vi "Logging.vi"(8 "error in (no error)":errorcluster, 11 "Node Ptr":T2 format="%.0x") -> (0 "error out":errorcluster)   [LabVIEW 2020, in "Ballard MIL-STD-1553 System Explorer.lvlib" / "Implementation.lvlib"]
uses:
  Implementation.lvlib
  <vilib>/NI VeriStand/Custom Device API/Custom Device Item Ref.ctl
  Shared/Data Word Format.ctl
  <vilib>/NI VeriStand/Custom Device API/Custom Device API.lvlib
  Scripting/Ballard MIL-STD-1553 Scripting.lvlib
panel:
  in  "Data Word Format":T1
  in  "Timestamp Filename":bool
  in  "File Name":string
  out "Example Log File Path":string
  in  "Enable Logging":bool
  in  "Log Directory":string
  in  "SHDocVw.IWebBrowser":refnum<k7>(container)
  in  "General Header":cluster{"Section Name":string}={"Section Name"="Ballard MIL-STD-1553 - Logging"}
  in  "Description":string
  out "Name":string
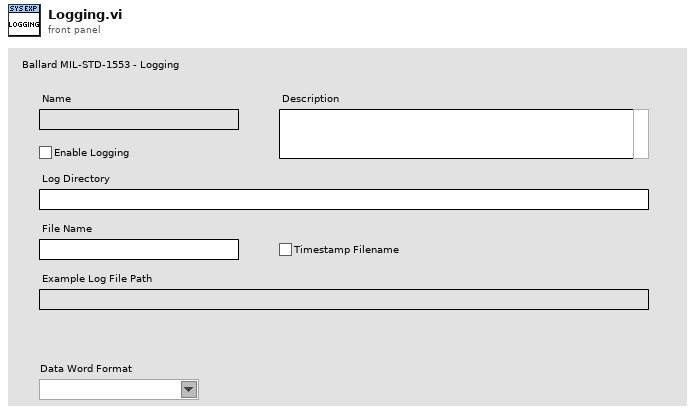
[diagram p1: front panel]
types:
  T1 = typedef "Data Word Format.ctl" = string
  T2 = typedef "Custom Device API.lvlib/Custom Device Item Ref.ctl" = u64
  T3 = typedef "Custom Device API.lvlib/Custom Device Item Info.ctl" = cluster{"Name":string, "Is Channel":bool, "GUID":string, "Is Waveform":bool}
  T4 = typedef "Custom Device API.lvlib/Custom Device Commands.ctl" = enum16{"Default", "Item renamed", "Shutdown", "Dynamic button pressed"}
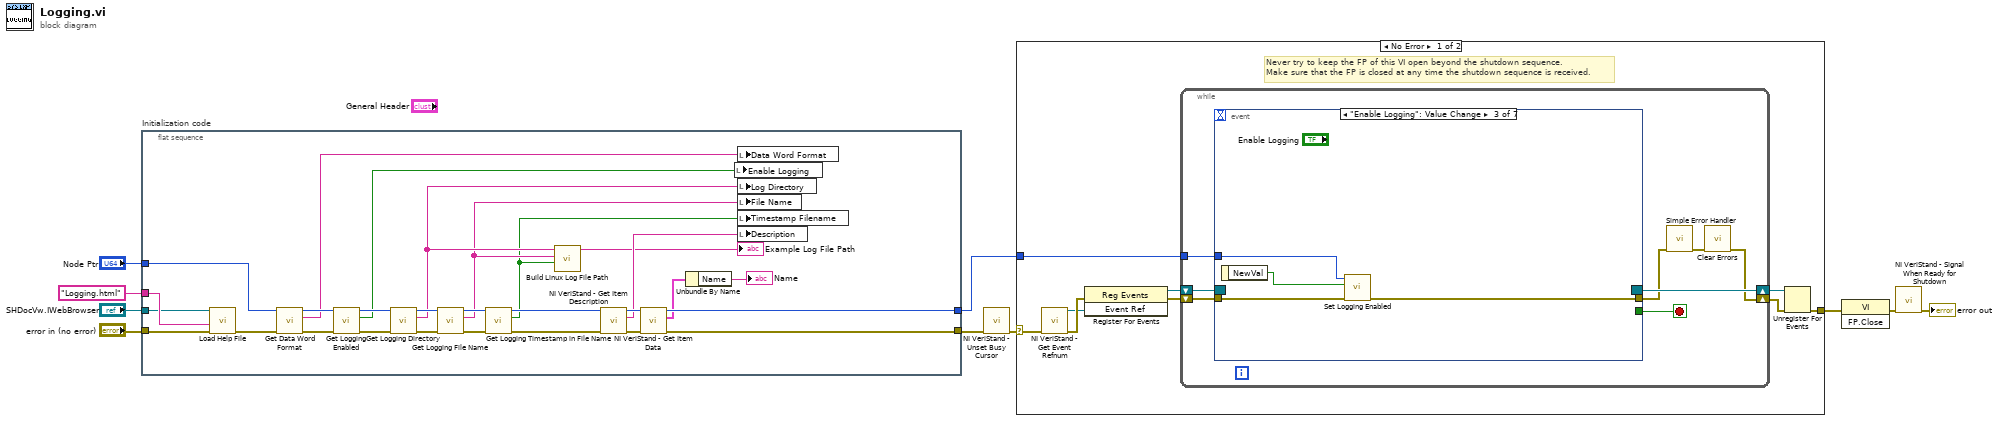
[diagram p0: block diagram]
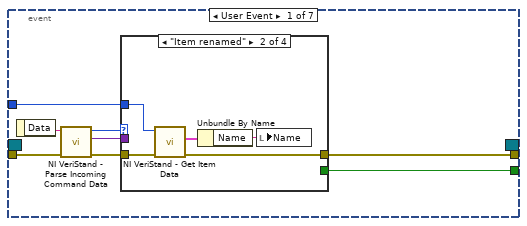
[diagram p2: hidden frame]
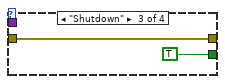
[diagram p4: hidden frame]
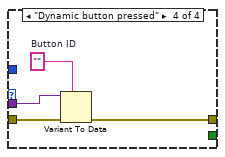
[diagram p5: hidden frame]
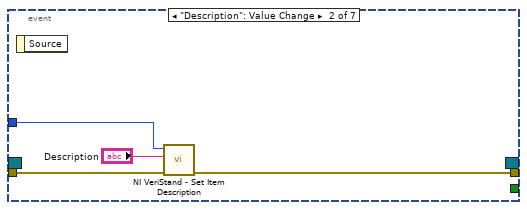
[diagram p6: hidden frame]
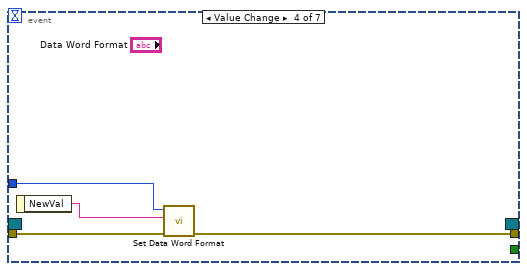
[diagram p7: hidden frame]
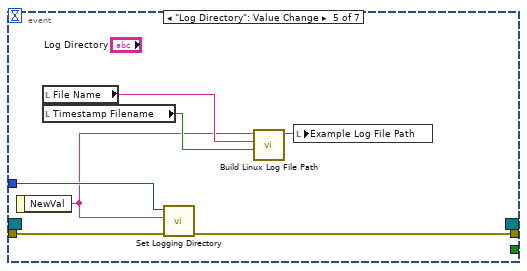
[diagram p8: hidden frame]
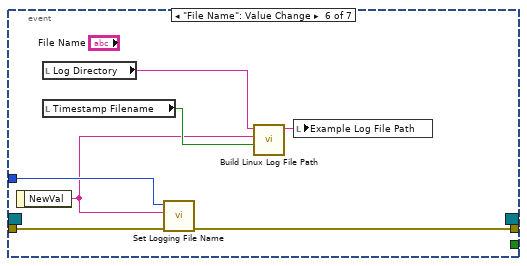
[diagram p9: hidden frame]
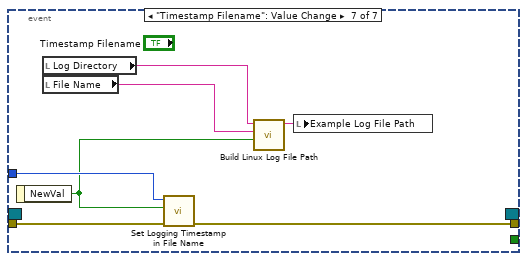
[diagram p10: hidden frame]
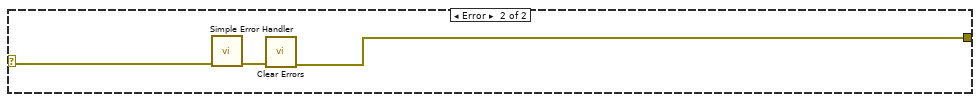
[diagram p11: hidden frame]
diagram:
  n1 = flat-sequence "Initialization code" {
    tunnel: "error in (no error)" -> [w32]
    tunnel: "Node Ptr" -> [w23]
    tunnel: [w34] -> w6
    tunnel: [w38] -> w3
    tunnel: "SHDocVw.IWebBrowser" -> [w30]
    tunnel: "Logging.html" ("CD_CHM_Section") -> [w31]
    frame #0 {
      n2 = call "Load Help File.vi"("error in (no error)"=w32, "HTML File to Load"=w31, "Browser"=w30) -> ("error out"=w28:errorcluster)  [unwired: 8 in]
      n3 = call "Get Data Word Format.vi"("error in"=w28, "logging in"=w23) -> ("error out"=w24:errorcluster, "data word format"=w21:T1, "logging out"=w22:T2)  [unwired: 7 in]
      n4 = call "Get Logging Enabled.vi"("error in"=w24, "logging in"=w22) -> ("error out"=w27:errorcluster, "logging enabled"=w25:bool, "logging out"=w26:T2)  [unwired: 7 in]
      n5 = call "Get Logging Directory.vi"("error in"=w27, "logging in"=w26) -> ("error out"=w19:errorcluster, "directory"=w13:string, "logging out"=w20:T2)  [unwired: 7 in]
      n6 = call "Get Logging File Name.vi"("error in"=w19, "logging in"=w20) -> ("error out"=w18:errorcluster, "file name"=w12:string, "logging out"=w17:T2)  [unwired: 7 in]
      n7 = call "Get Logging Timestamp in File Name.vi"("error in"=w18, "logging in"=w17) -> ("error out"=w16:errorcluster, "timestamp in file name"=w11:bool, "logging out"=w15:T2)  [unwired: 7 in]
      n8 = call "Build Linux Log File Path.vi"("Timestamp"=w11, "Name"=w12, "Log File Directory"=w13) -> ("Log File Path"=→"Example Log File Path":string)  [unwired: 7 in, 1 out]
      n9 = call <vilib>:"NI VeriStand - Get Item Description.vi"("error in (no error)"=w16, "Item Ref in"=w15) -> ("error out"=w36:errorcluster, "Description"=w33:string, "Item Ref out"=w37:T2)  [unwired: 7 out]
      n10 = call <vilib>:"NI VeriStand - Get Item Data.vi"("error in (no error)"=w36, "Item Ref in"=w37) -> ("error out"=w34:errorcluster, "Item Info"=w35:T3, "Item Ref out"=w38:T2)  [unwired: 7 out]
      n11 = Unbundle By Name(w35) -> ("Name"=→"Name":string)
      n12 = local write "Enable Logging"(w25) -> ()
      n13 = local write "Data Word Format"(w21) -> ()
      n14 = local write "Log Directory"(w13) -> ()
      n15 = local write "File Name"(w12) -> ()
      n16 = local write "Timestamp Filename"(w11) -> ()
      n17 = local write "Description"(w33) -> ()
    }
  }
  n18 = call <vilib>:"NI VeriStand - Unset Busy Cursor.vi"("error in (no error)"=w6) -> ("error out"=w5:errorcluster)  [unwired: 10 out]
  n19 = case shown="No Error" w5 {
    selector: w5 -> [w39 w111]
    tunnel: [w44 w109] -> w10
    tunnel: w3 -> [w40 _]
    frame No Error {
      # "Never try to keep the FP of this VI open beyond the shutdown sequence.\nMake sure that the FP is closed at any time the shutdown sequence is received."
      n20 = call <vilib>:"NI VeriStand - Get Event Refnum.vi"("error in (no error)"=w39) -> ("error out"=w47:errorcluster, "Event Ref"=w43:refnum<user-event>)  [unwired: 9 out]
      n21 = register-events(error in=w47, w43) -> (reference out=w41:refnum<event-registration>, error out=w42:errorcluster)  [unwired: 1 in]
      n22 = while {
        tunnel: w40 -> [w51]
        shift-right: [w48] -> w45
        shift-left: w42 -> [w54]
        shift-right: [w55] -> w46
        shift-left: w41 -> [w53]
        stop <- w52 stop-if-true
        n23 = event shown="[2] \"Enable Logging\": Value Change" {
          selector: w53 -> [_ _ _ _ _ _ _]
          dyn-events: [_ _ _ _ _ _ _] -> w55
          timeout: _ -> [_ _ _ _ _ _ _]
          tunnel: w54 -> [w63 w78 w83 w86 w94 w101 w108]
          tunnel: [w59 _ _ _ _ _ _] -> w52
          tunnel: [w58 w77 w82 w87 w92 w100 w107] -> w50
          tunnel: w51 -> [w57 w79 w81 w85 w93 w99 w106]
          event User Event {
            n24 = event-data() -> ("Data"=w62:string)  [unwired: 1 out]
            n25 = call <vilib>:"NI VeriStand - Parse Incoming Command Data.vi"("error in (no error)"=w63, "Incoming data"=w62) -> ("error out"=w61:errorcluster, "Outgoing data"=w56:variant, "Action"=w60:T4)  [unwired: 7 out]
            n26 = case shown="\"Item renamed\"" w60 {
              tunnel: w61 -> [w64 w69 w70 w75]
              tunnel: [_ _ TRUE _] -> w59
              tunnel: [w64 w66 w70 w72] -> w58
              tunnel: w57 -> [_ w68 _ _]
              tunnel: w56 -> [_ _ _ w74]
              frame "Default", Default {
              }
              frame "Item renamed" {
                n27 = call <vilib>:"NI VeriStand - Get Item Data.vi"("error in (no error)"=w69, "Item Ref in"=w68) -> ("error out"=w66:errorcluster, "Item Info"=w67:T3)  [unwired: 8 out]
                n28 = Unbundle By Name(w67) -> ("Name"=w65:string)
                n29 = local write "Name"(w65) -> ()
              }
              frame "Shutdown" {
              }
              frame "Dynamic button pressed" {
                w73 = ""  # Button ID
                n30 = Variant To Data(error in=w75, type=w73, Variant=w74) -> (error out=w72:errorcluster)  [unwired: 1 out]
              }
            }
          }
          event "Description": Value Change {
            n31 = event-data() -> ()  [unwired: 2 out]
            n32 = call <vilib>:"NI VeriStand - Set Item Description.vi"("error in (no error)"=w78, "Description"="Description", "Item Ref in"=w79) -> ("error out"=w77:errorcluster)  [unwired: 8 out]
          }
          event "Enable Logging": Value Change {
            n33 = event-data() -> ("NewVal"=w80:bool)  [unwired: 1 out]
            n34 = call "Set Logging Enabled.vi"("error in"=w83, "logging enabled"=w80, "logging in"=w81) -> ("error out"=w82:errorcluster)  [unwired: 7 in, 1 out]
          }
          event Value Change {
            n35 = event-data() -> ("NewVal"=w84:T1)  [unwired: 1 out]
            n36 = call "Set Data Word Format.vi"("error in"=w86, "data word format"=w84, "logging in"=w85) -> ("error out"=w87:errorcluster)  [unwired: 7 in, 1 out]
          }
          event "Log Directory": Value Change {
            n37 = event-data() -> ("NewVal"=w88:string)  [unwired: 1 out]
            n38 = local read "File Name"() -> (w90:string)
            n39 = local read "Timestamp Filename"() -> (w89:bool)
            n40 = call "Set Logging Directory.vi"("error in"=w94, "directory"=w88, "logging in"=w93) -> ("error out"=w92:errorcluster)  [unwired: 6 in, 1 out]
            n41 = call "Build Linux Log File Path.vi"("Timestamp"=w89, "Name"=w90, "Log File Directory"=w88) -> ("Log File Path"=w91:string)  [unwired: 7 in, 1 out]
            n42 = local write "Example Log File Path"(w91) -> ()
          }
          event "File Name": Value Change {
            n43 = event-data() -> ("NewVal"=w95:string)  [unwired: 1 out]
            n44 = local read "Log Directory"() -> (w97:string)
            n45 = local read "Timestamp Filename"() -> (w96:bool)
            n46 = call "Set Logging File Name.vi"("error in"=w101, "file name"=w95, "logging in"=w99) -> ("error out"=w100:errorcluster)  [unwired: 6 in, 1 out]
            n47 = call "Build Linux Log File Path.vi"("Timestamp"=w96, "Name"=w95, "Log File Directory"=w97) -> ("Log File Path"=w98:string)  [unwired: 7 in, 1 out]
            n48 = local write "Example Log File Path"(w98) -> ()
          }
          event "Timestamp Filename": Value Change {
            n49 = event-data() -> ("NewVal"=w104:bool)  [unwired: 1 out]
            n50 = local read "Log Directory"() -> (w103:string)
            n51 = local read "File Name"() -> (w102:string)
            n52 = call "Set Logging Timestamp in File Name.vi"("error in"=w108, "timestamp in file name"=w104, "logging in"=w106) -> ("error out"=w107:errorcluster)  [unwired: 7 in, 1 out]
            n53 = call "Build Linux Log File Path.vi"("Timestamp"=w104, "Name"=w102, "Log File Directory"=w103) -> ("Log File Path"=w105:string)  [unwired: 7 in, 1 out]
            n54 = local write "Example Log File Path"(w105) -> ()
          }
        }
        n55 = call <vilib>:"Simple Error Handler.vi"("error in (no error)"=w50) -> ("error out"=w49:errorcluster)  [unwired: 1 in, 7 out]
        n56 = call <vilib>:"Clear Errors.vi"("error in (no error)"=w49) -> ("error out"=w48:errorcluster)  [unwired: 1 in, 5 out]
      }
      n57 = Unregister For Events(event registration refnum=w46, error in=w45) -> (error out=w44:errorcluster)
    }
    frame Error {
      n58 = call <vilib>:"Simple Error Handler.vi"("error in (no error)"=w111) -> ("error out"=w110:errorcluster)  [unwired: 1 in, 7 out]
      n59 = call <vilib>:"Clear Errors.vi"("error in (no error)"=w110) -> ("error out"=w109:errorcluster)  [unwired: 1 in, 5 out]
    }
  }
  n60 = invoke class="VI" method="FP.Close"(error in=w10) -> (error out=w9:errorcluster)  [unwired: 2 in, 2 out]
  n61 = call <vilib>:"NI VeriStand - Signal When Ready for Shutdown.vi"("error in (no error)"=w9) -> ("error out"=→"error out":errorcluster)  [unwired: 10 out]
